vi "getHealthAndStatus.vi"(11 "Model in":refnum<class "Model.lvclass">) -> (2 "HealthAndStatus":refnum<class "RTHealthAndStatus.lvclass">, 3 "Model out":refnum<class "Model.lvclass">)   [LabVIEW 2016, in "Model.lvclass"]
uses:
  Model.lvclass
  Common_RT_HealthAndStatus/RTHealthAndStatus/RTHealthAndStatus.lvclass
  Model.lvclass/Model.ctl
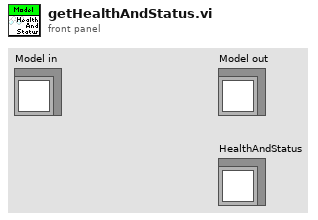
[diagram p1: front panel]
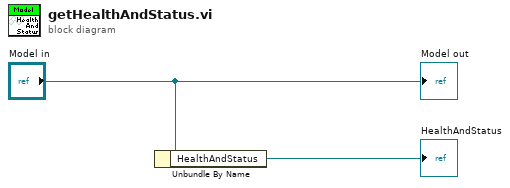
[diagram p0: block diagram]
diagram:
  n1 = Unbundle By Name("Model in") -> ("HealthAndStatus"=→"HealthAndStatus":refnum<class "RTHealthAndStatus.lvclass">)
  "Model out" <- "Model in"
